vi "Create.vi"(8 "error in (no error)":errorcluster, 11 "Core Channel User Interface in":refnum<class "Core Channel User Interface.lvclass">) -> (0 "error out":errorcluster, 3 "Core Channel User Interface out":refnum<class "Core Channel User Interface.lvclass">)   [LabVIEW 2017, in "DSF Core.lvlib" / "Core Channel User Interface.lvclass"]
uses:
  Core Channel User Interface.lvclass
  C:/Git/DSF/Core/Classes/User Interface/User Interface.lvclass
  Configuration/Core/Channel/Core Channels Configuration.lvclass
  C:/Git/DSF/Core/Classes/Configuration/Configuration.lvclass
  User Interface.vi
  User Interface.lvclass
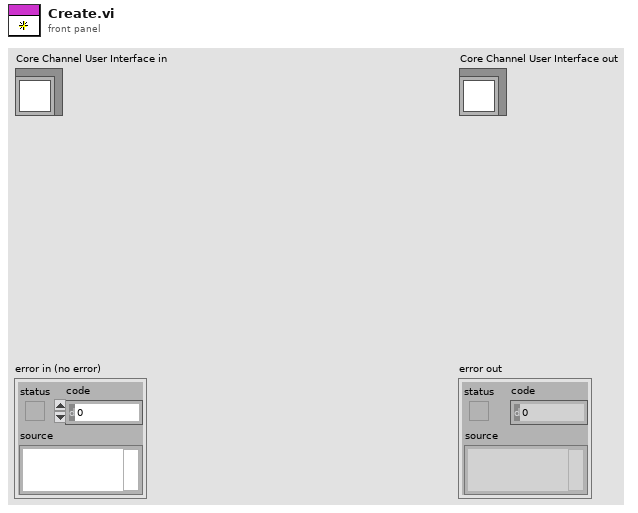
[diagram p1: front panel]
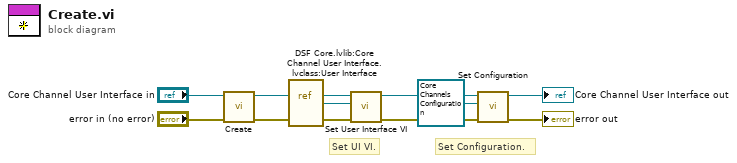
[diagram p0: block diagram]
diagram:
  # "Set Configuration."
  # "Set UI VI."
  n1 = call-parent "Create.vi"("error in (no error)"="error in (no error)", "User Interface in"="Core Channel User Interface in") -> ("error out"=w8:errorcluster, "User Interface out"=w7:refnum<class "Core Channel User Interface.lvclass">)  [unwired: 8 in]
  n2 = vi-ref "DSF Core.lvlib:Core Channel User Interface.lvclass:User Interface.vi"() -> (w1:refnum<vi>)
  n3 = call "Set User Interface VI.vi"("error in (no error)"=w8, "vi"=w1, "User Interface in"=w7) -> ("error out"=w6:errorcluster, "User Interface out"=w5:refnum<class "Core Channel User Interface.lvclass">)  [unwired: 7 in]
  n4 = call "Set Configuration.vi"("error in (no error)"=w6, "configuration"=refnum<class "Core Channels Configuration.lvclass"> refnum ("DSF Core.lvlib:Core Channels Configuration.lvclass"), "User Interface in"=w5) -> ("error out"=→"error out":errorcluster, "User Interface out"=→"Core Channel User Interface out":refnum<class "Core Channel User Interface.lvclass">)  [unwired: 7 in]
